vi "Get Type Specializations.vi"(8 "error in (no error)":errorcluster) -> (0 "error out":errorcluster, 2 "Type Specializations":T1[](array[typedef]))   [LabVIEW 2020, in "MeasurementLink Measurement Template.lvlib"]
uses:
  MeasurementLink Measurement Template.lvlib
  <vilib>/MeasurementLink/MeasurementLink Measurement Server/Helpers/TypeDefs/Key.ctl
  <vilib>/MeasurementLink/MeasurementLink Measurement Server/Helpers/TypeDefs/Type Specialization.ctl
  <vilib>/MeasurementLink/MeasurementLink Measurement Server/Helpers/TypeDefs/Parameter Type Specialization.ctl
  Runtime/MeasurementLink Measurement Server/MeasurementLink Measurement Server.lvlib
panel:
  in  "Enum":enum16{"Hello", "World", "Foo", "Bar"}(ring)
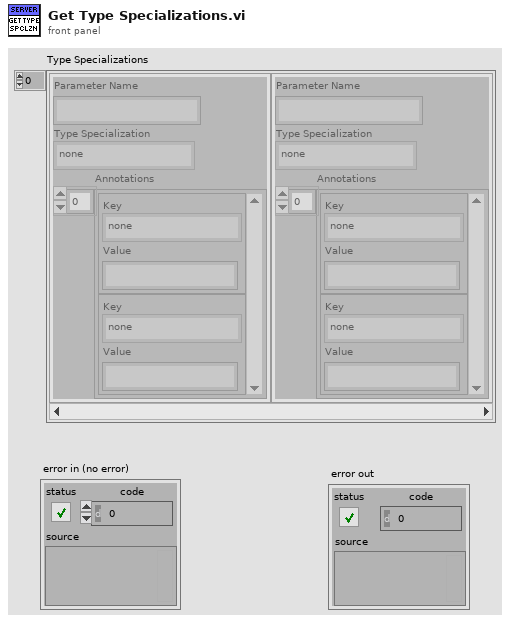
[diagram p1: front panel]
types:
  T1 = typedef "MeasurementLink Measurement Server.lvlib/Parameter Type Specialization.ctl" = cluster{"Parameter Name":string, "Type Specialization":T2, "Annotations":cluster{"Key":T3, "Value":string}[]}
  T2 = typedef "MeasurementLink Measurement Server.lvlib/Type Specialization.ctl" = enum16{"none", "pin", "path"}
  T3 = typedef "MeasurementLink Measurement Server.lvlib/Key.ctl" = enum16{"none", "pin.instrument_type"}
  T4 = typedef "MeasurementLink Measurement Server.lvlib/Parameter Type Specialization.ctl" = cluster{"Parameter Name":string, "Type Specialization":T5, "Annotations":cluster{"Key":T6, "Value":string}[]}
  T5 = typedef "MeasurementLink Measurement Server.lvlib/Type Specialization.ctl" = enum16{"none", "pin", "path", "enum"}
  T6 = typedef "MeasurementLink Measurement Server.lvlib/Type Specialization Key.ctl" = enum16{"none", "pin.instrument_type", "enum.values"}
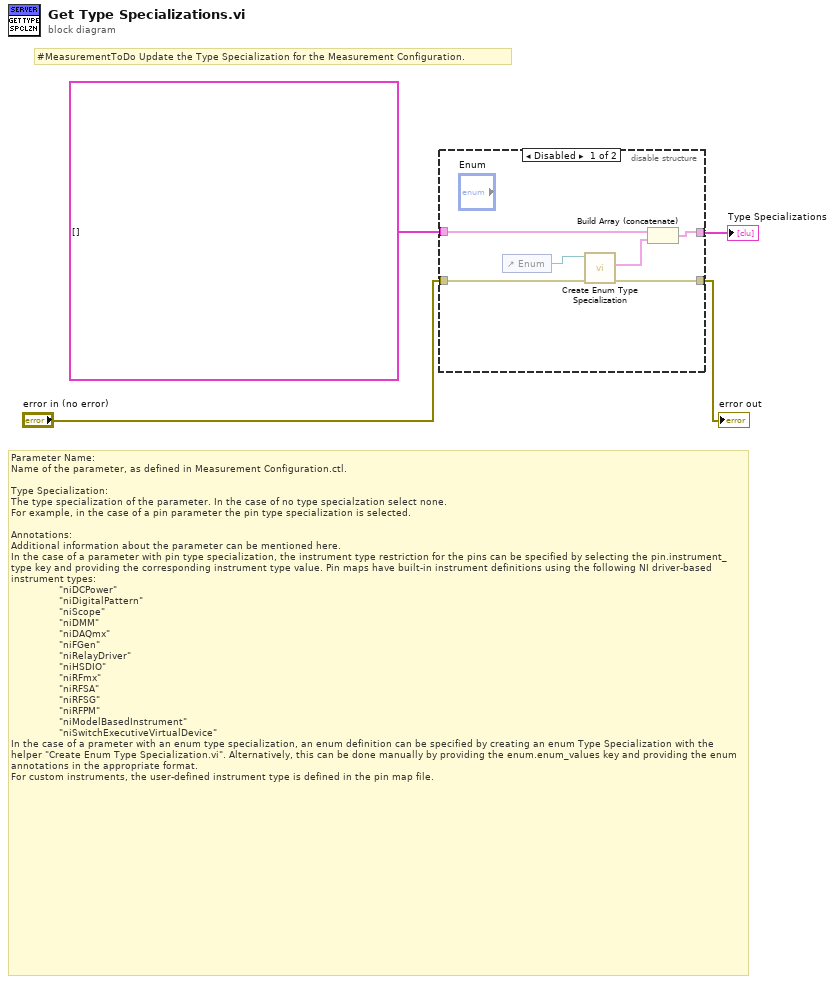
[diagram p0: block diagram]
diagram:
  # "Parameter Name: \nName of the parameter, as defined in Measurement Configuration.ctl.\n\nType Specialization: \nThe type specialization of the parameter. In the case of no type specialzation select none. \nFor example, in the case of a pin parameter the pin type specialization is selected.\n\nAnnotations:\nAdditional information about the parameter can be mentioned here.\nIn the case of a parameter with pin type specialization, the instrument type restriction for the pins can be specified by selecting the pin.instrument_type key and providing the corresponding instrument type value. Pin maps have built-in instrument definitions using the following NI driver-based instrument types:\n                \"niDCPower\"\n                \"niDigitalPattern\"\n                \"niScope\"\n                \"niDMM\"\n                \"niDAQmx\"\n                \"niFGen\"\n                \"niRelayDriver\"\n                \"niHSDIO\"\n                \"niRFmx\"\n                \"niRFSA\"\n                \"niRFSG\"\n                \"niRFPM\"\n                \"niModelBasedInstrument\"\n                \"niSwitchExecutiveVirtualDevice\"\nIn the case of a prameter with an enum type specialization, an enum definition can be specified by creating an enum Type Specialization with the helper \"Create Enum Type Specialization.vi\". Alternatively, this can be done manually by providing the enum.enum_values key and providing the enum annotations in the appropriate format.\nFor custom instruments, the user-defined instrument type is defined in the pin map file."
  # "#MeasurementToDo Update the Type Specialization for the Measurement Configuration."
  n1 = disable-structure shown="Disabled" {
    disable-tunnel: T1[] [] -> [w10 w11]
    disable-tunnel: [w8 w11] -> w3
    disable-tunnel: [w7 _] -> w2
    disable-tunnel: "error in (no error)" -> [w6 _]
    frame Disabled {
      n2 = control-ref of="Enum"() -> (w5:refnum<vi>)
      n3 = call "Create Enum Type Specialization.vi"("error in (no error)"=w6, "Enum Reference"=w5) -> ("error out"=w7:errorcluster, "Parameter Type Specialization Output"=w9:T4)  [unwired: 6 in, 1 out]
      n4 = Build Array (concatenate)(w10, w9) -> (w8:T4[])
    }
    frame Enabled {
    }
  }
  "Type Specializations" <- w3
  "error out" <- w2
